vi "Photoresistor Edge Detection.vi"() -> ()   [LabVIEW 2022 SP3]
uses:
  <vilib>/MakerHub/LINX/Public/Utilities/Open Serial.vi
  <vilib>/MakerHub/LINX/LMH-LINX.lvlib
panel:
  out "Falling Edge":bool
  out "Falling Edge":i16(graph)
  out "Rising Edge":i16(graph)
  out "Rising Edge":bool
  in  "Threshold":dbl
  out "Digitized Signal":i16(graph)
  in  "stop":bool
  in  "AI Channel":u8
  in  "Serial Port":refnum<visa-resource-name>="N/A"
  out "Photoresistor Readings":dbl(graph)
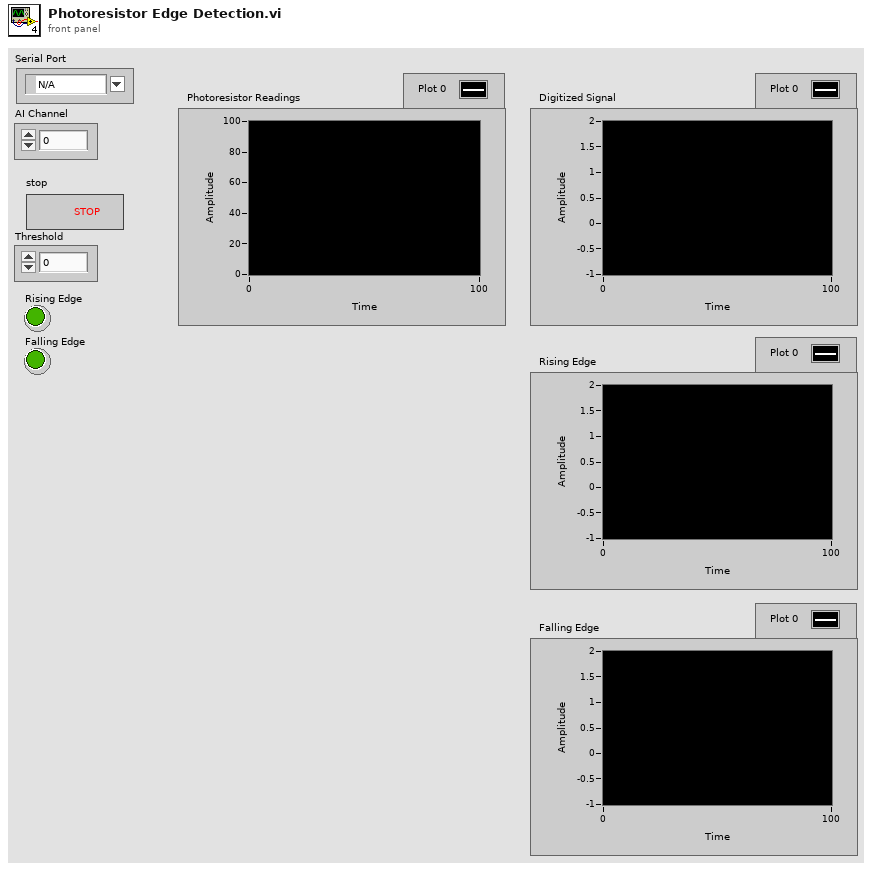
[diagram p1: front panel]
types:
  T1 = typedef "LMH-LINX.lvlib/LINX Ref.ctl" = cluster{"IO":T2, "Interface":T3, "LINX Device Config":T4}
  T2 = typedef "LMH-LINX.lvlib/Platform.ctl" = enum16{"Remote", "Local"}
  T3 = typedef "LMH-LINX.lvlib/Interface.ctl" = enum16{"Serial", "TCP"}
  T4 = typedef "LMH-LINX.lvlib/Device.lvlib/LINX Device Config.ctl" = cluster{"Interface":T3, "COM Port":refnum<visa-resource-name>, "TCP Configuration":T5, "Device Family":u8, "Device ID":u8, "Device Name":string, "TCP Ref":refnum<k5>, "Channels":T6}
  T5 = typedef "LMH-LINX.lvlib/Device.lvlib/TCP Config.ctl" = cluster{"IP Address":string, "Port":u16}
  T6 = typedef "LMH-LINX.lvlib/Channels.ctl" = cluster{"DI":u8[], "DO":u8[], "AI":u8[], "AO":u8[], "PWM":u8[], "QE":u8[], "UART":u8[], "I2C 2":u8[], "SPI":u8[], "CAN":u8[], "Servo":u8[], "AI Ref (V)":dbl, "AI Resolution (Bits)":u8, "AO Ref (V)":dbl, "AO Resolution (Bits)":u8}
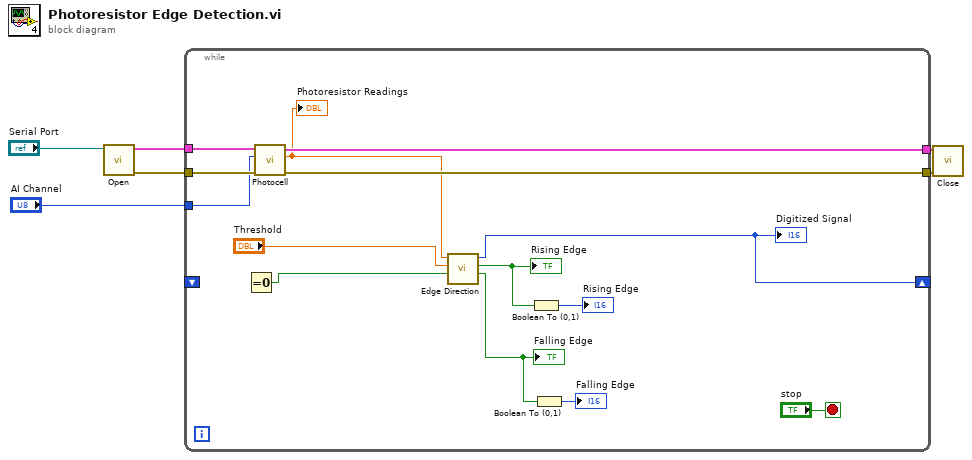
[diagram p0: block diagram]
diagram:
  n1 = call-poly <vilib>:"Open.vi"("Serial Port"="Serial Port") -> ("Error Out"=w5:errorcluster, "LINX Resource"=w6:T1)  [unwired: 8 in, 1 out]
  n2 = while {
    tunnel: w6 -> [w20]
    tunnel: w5 -> [w19]
    tunnel: [w18] -> w4
    tunnel: [w17] -> w3
    tunnel: "AI Channel" -> [w16]
    shift-right: [w7] -> _
    shift-left: _ -> [_]
    stop <- "stop" stop-if-true
    n3 = Equal To 0?() -> (x = 0?=w12:bool)  [unwired: 1 in]
    n4 = call <vilib>:"Photocell.vi"("Error In"=w19, "AI Channel"=w16, "LINX Resource"=w20) -> ("Error Out"=w17:errorcluster, "Value (0-100)"=w13:dbl, "LINX Resource"=w18:T1)  [unwired: 6 in]
    "Photoresistor Readings" <- w13
    n5 = call "Edge Direction.vi"("Previous Value"=w12, "Threshold"="Threshold", "Analog Input"=w13) -> ("Falling Edge"=w10:bool, "Rising Edge"=w8:bool, "Digitized"=w7:i16)  [unwired: 6 in]
    "Digitized Signal" <- w7
    "Rising Edge" <- w8
    "Falling Edge" <- w10
    n6 = Boolean To (0,1)(Boolean=w8) -> (0, 1=→"Rising Edge":i16)
    n7 = Boolean To (0,1)(Boolean=w10) -> (0, 1=→"Falling Edge":i16)
  }
  n8 = call <vilib>:"Close.vi"("Error In"=w3, "LINX Resource"=w4) -> ()  [unwired: 9 in, 1 out]
